vi "flush_TMC_buffer.vi"(6 "Echo Mode":i32, 7 "Ignore/Clear Error (t/f)":bool, 8 "error in":errorcluster={"status"=FALSE, "code"=1073676294, "source"="VISA Read in write_read.vi"}, 11 "ComPort":refnum<visa-resource-name>="COM3") -> (0 "error out":errorcluster={"status"=FALSE, "code"=1073676294, "source"="VISA Read in write_read.vi"}, 2 "Firmware Version":string, 3 "VISA ressource out":refnum<visa-resource-name>)   [LabVIEW 2018]
uses:
  MCode_LV_86/Set Parameter.ctl
panel:
  out "Error Value 3":string
  out "Error Value 2":string
  out "Error Value 1":string
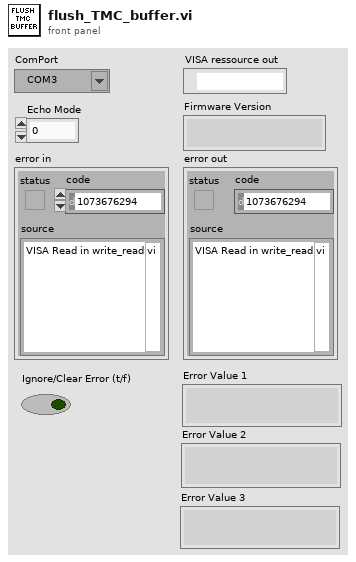
[diagram p1: front panel]
types:
  T1 = typedef "Set Parameter.ctl" = enum16{"Acceleration (A)", "Baud Rate (BD)", "Counter 1 (C1)", "Counter 2 (C2)", "Control C Software Reset (CE)", "Check Sum Enable (CK)", "Clock Mode (CM)", "Clock Mode Ratio (CR)", "Clock Mode Out Step Width (CW)", "Deceleration (D)", "Digital Filtering, Input 1 (D1)", "Digital Filtering, Input 2 (D2)", "Digital Filtering, Input 3 (D3)", "Digital Filtering, Input 4 (D4)", "Digital Filtering, Input 5 (D5)", "Digital Filtering, Input 9 (D9)", "Digital Filtering, Input 10 (D10)", "Digital Filtering, Input 11 (D11)", "Digital Filtering, Input 12 (D12)", "Deadband (DB)", "Decrement Variable (DC)", "Enable/Disable Drive (DE)", "Device Name (DN)", "End Program Execution (E)", "Encoder Function Enable (EE)", "Error Flag (EF)", "Encoder Lines (EL)", "Echo Mode (EM)", "Error Value (ER)", "Escape (ES)", "Execute Program at Address (EX)", "Firmware Version (VR)", "Hold (H)", "Hold Current (HC)", "Hold Current Delay Time (HI)", "Home to Encoder Index (HM)", "Home to Home Switch (HT)", "Increment Variable (IC)", "Initialize Parameters to NVM (IP)", "Input into Variable (IV)", "Jog Enable (JE)", "Limit Stop Mode (LM)", "Move Absolute (MA)", "Move Relative (MR)", "MicroStepping Select (MS)", "Motor Settling Delay Time (MT)", "Moving [Flag] (MV)", "Output 1 (O1)", "Output 2 (O2)", "Output 3 (O3)", "Output 4 (O4)", "Output 9 (O9)", "Output 10 (O10)", "Output 11 (O11)", "Output 12 (O12)", "Output High Byte (9-12) (OH)", "Output Low Byte (1-4) (OL)", "Output Total (1-4 and 9-12) (OT)", "Position (P)", "Position Maintenance (PM)", "Party Mode (PY)", "Register 1 (R1)", "Register 2 (R2)", "Register 3 (R3)", "Register 4 (R4)", "Reset Error(\\03)", "Run Current (RC)", "Stall Factor (SF)", "Slew (SL)", "Stall Mode Set (SM)", "Upgrade Firmware (UG)", "Velocity Initial (VI)", "Velocity Maximum (VM)", "Current1 (I1)", "Current2 (I2)", "Current3 (I3)", "Current4 (I4)", "Current5 (I5)", "Current6 (I6)", "Save (S)"}
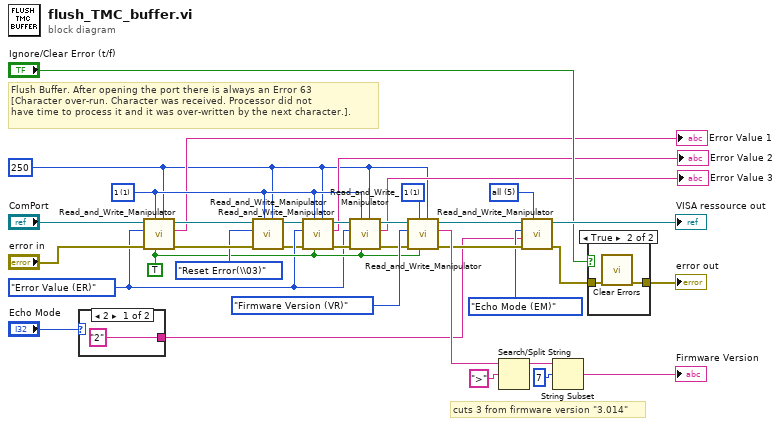
[diagram p0: block diagram]
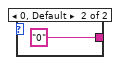
[diagram p3: hidden frame]
diagram:
  w2 = u16 1 items=["none", "1", "2", "3", "4", "all"] ("Motor")
  w9 = u16 5 items=["none", "1", "2", "3", "4", "all"] ("Motor")
  w1 = 250
  w25 = TRUE ("Print?")
  w24 = Set_Parameter."Error Value (ER)" ("Command")
  w23 = u16 1 items=["none", "1", "2", "3", "4", "all"] ("Motor")
  # "cuts 3 from firmware version \"3.014\""
  # "Flush Buffer. After opening the port there is always an Error 63\n[Character over-run. Character was received. Processor did not\nhave time to process it and it was over-written by the next character.]."
  n1 = case shown="2" "Echo Mode" {
    tunnel: ["2" ("Value") "0" ("Value")] -> w11
    frame 2 {
    }
    frame 0, Default {
    }
  }
  n2 = call "Read_and_Write_Manipulator.vi"("additional waiting time (0)"=w1, "Print?"=w25, "Motor"=w23, "error in (no error)"="error in", "Command"=w24, "VISA resource name"="ComPort") -> ("error out"=w31:errorcluster, "Answer"=→"Error Value 1":string, "VISA ressource out"=w33:refnum<visa-resource-name>)  [unwired: 1 in, 2 out]
  n3 = call "Read_and_Write_Manipulator.vi"("additional waiting time (0)"=w1, "Motor"=w23, "error in (no error)"=w31, "Command"=Set_Parameter."Reset Error(\\03)", "VISA resource name"=w33) -> ("error out"=w16:errorcluster, "VISA ressource out"=w28:refnum<visa-resource-name>)  [unwired: 2 in, 3 out]
  n4 = call "Read_and_Write_Manipulator.vi"("additional waiting time (0)"=w1, "Print?"=w25, "Motor"=w23, "error in (no error)"=w16, "Command"=w24, "VISA resource name"=w28) -> ("error out"=w26:errorcluster, "Answer"=→"Error Value 2":string, "VISA ressource out"=w27:refnum<visa-resource-name>)  [unwired: 1 in, 2 out]
  n5 = call "Read_and_Write_Manipulator.vi"("additional waiting time (0)"=w1, "Print?"=w25, "Motor"=w23, "error in (no error)"=w26, "Command"=w24, "VISA resource name"=w27) -> ("error out"=w22:errorcluster, "Answer"=→"Error Value 3":string, "VISA ressource out"=w32:refnum<visa-resource-name>)  [unwired: 1 in, 2 out]
  n6 = call "Read_and_Write_Manipulator.vi"("additional waiting time (0)"=w1, "Print?"=w25, "Motor"=w2, "error in (no error)"=w22, "Command"=Set_Parameter."Firmware Version (VR)", "VISA resource name"=w32) -> ("error out"=w14:errorcluster, "Answer"=w20:string, "VISA ressource out"=w15:refnum<visa-resource-name>)  [unwired: 1 in, 2 out]
  n7 = Search/Split String(string=w20, search string/char (-)=">") -> (substring before match=w19:string)  [unwired: 1 in, 2 out]
  n8 = call "Read_and_Write_Manipulator.vi"("Motor"=w9, "error in (no error)"=w14, "Value"=w11, "Command"=Set_Parameter."Echo Mode (EM)", "VISA resource name"=w15) -> ("error out"=w8:errorcluster, "VISA ressource out"=→"VISA ressource out":refnum<visa-resource-name>)  [unwired: 2 in, 3 out]
  n9 = String Subset(string=w19, offset (0)=7) -> (substring=→"Firmware Version":string)  [unwired: 1 in]
  n10 = case shown="True" "Ignore/Clear Error (t/f)" {
    tunnel: w8 -> [w38 w40]
    tunnel: [w38 w39] -> w7
    frame False {
    }
    frame True {
      n11 = call <vilib>:"Clear Errors.vi"("error in (no error)"=w40) -> ("error out"=w39:errorcluster)  [unwired: 5 in, 1 out]
    }
  }
  "error out" <- w7
